vi "SimpleRobot_Dynamics_RevA.vi"(0 "x0":dbl, 1 "Wind Speed":dbl, 2 "Wind Direction":dbl, 5 "x1":dbl, 7 "y0":dbl, 9 "y1":dbl, 11 "Velocity":dbl, 12 "Direction":dbl, 13 "DeltaT (timestep)":dbl) -> (4 "x 2":dbl, 6 "y 2":dbl, 10 "Direction 2":dbl, 15 "Boat Velocity Out":dbl)   [LabVIEW 2012]
doc: "This subVI produces simple simulated robot dynamics.\nYou will need to replace it with a better simulation of your robot's dynamics"
panel:
  out "atan2(y,x)":dbl
  # "This VI calculates the Robot dynamics from frame to frame (one frame equals one time step)"
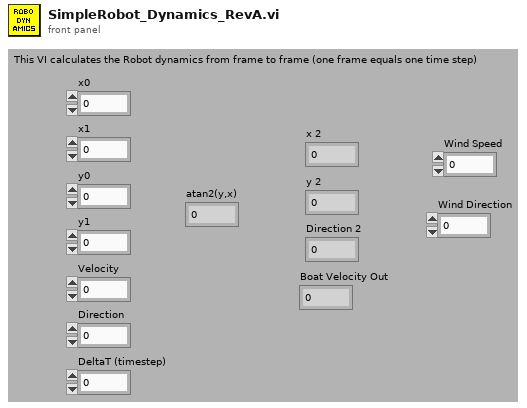
[diagram p1: front panel]
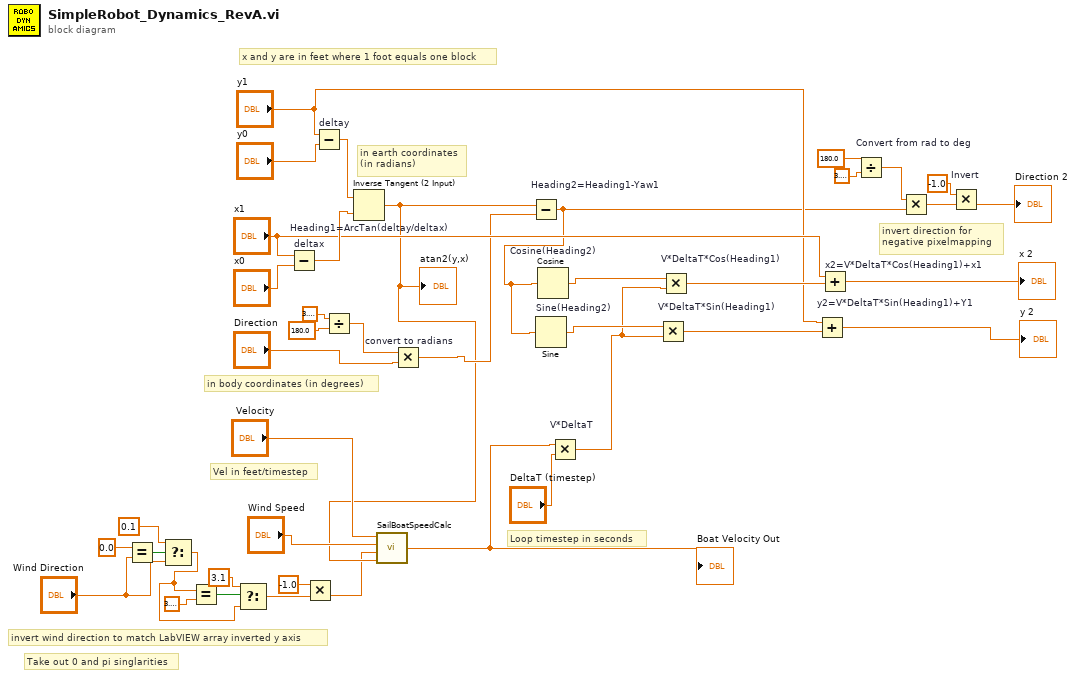
[diagram p0: block diagram]
diagram:
  # "Take out 0 and pi singlarities"
  # "invert wind direction to match LabVIEW array inverted y axis"
  # "invert direction for \nnegative pixelmapping"
  # "Loop timestep in seconds"
  # "x and y are in feet where 1 foot equals one block"
  # "Vel in feet/timestep"
  # "in earth coordinates\n(in radians)"
  # "in body coordinates (in degrees)"
  n1 = Equal?(x=0.0, y="Wind Direction") -> (x = y?=w9:bool)
  n2 = Select(t=0.1, s=w9, f="Wind Direction") -> (s? t:f=w1:dbl)
  n3 = Equal?(x=w1, y=3.141592653589793) -> (x = y?=w3:bool)
  n4 = Select(t=3.1, s=w3, f=w1) -> (s? t:f=w5:dbl)
  n5 = Subtract "deltax"(x="x1", y="x0") -> (x-y=w38:dbl)
  n6 = Multiply(x=-1.0, y=w5) -> (x*y=w11:dbl)
  n7 = Subtract "deltay"(x="y1", y="y0") -> (x-y=w39:dbl)
  n8 = Divide(x=3.141592653589793, y=180.0) -> (x/y=w27:dbl)
  n9 = Inverse Tangent (2 Input) "Heading1=ArcTan(deltay/deltax)"(1:w38, 2:w39) -> (0:w13:dbl)
  "atan2(y,x)" <- w13
  n10 = call "SailBoatSpeedCalc.vi"("Boat Direction"=w13, "Wind Direction (Rad global coordinates)"=w11, "Wind Speed"="Wind Speed", "Velocity Desired In"="Velocity") -> ("Boat Velocity Out"=w18:dbl)
  "Boat Velocity Out" <- w18
  n11 = Multiply "convert to radians"(x=w27, y="Direction") -> (x*y=w14:dbl)
  n12 = Subtract "Heading2=Heading1-Yaw1"(x=w13, y=w14) -> (x-y=w15:dbl)
  n13 = Sine "Sine(Heading2)"(x=w15) -> (sin(x)=w36:dbl)
  n14 = Cosine "Cosine(Heading2)"(x=w15) -> (cos(x)=w37:dbl)
  n15 = Multiply "V*DeltaT"(x=w18, y="DeltaT (timestep)") -> (x*y=w35:dbl)
  n16 = Multiply "V*DeltaT*Sin(Heading1)"(x=w36, y=w35) -> (x*y=w12:dbl)
  n17 = Multiply "V*DeltaT*Cos(Heading1)"(x=w37, y=w35) -> (x*y=w34:dbl)
  n18 = Add "y2=V*DeltaT*Sin(Heading1)+Y1"(x="y1", y=w12) -> (x+y=→"y 2":dbl)
  n19 = Add "x2=V*DeltaT*Cos(Heading1)+x1"(x="x1", y=w34) -> (x+y=→"x 2":dbl)
  n20 = Divide "Convert from rad to deg"(x=180.0, y=3.141592653589793) -> (x/y=w23:dbl)
  n21 = Multiply(x=w23, y=w15) -> (x*y=w20:dbl)
  n22 = Multiply "Invert"(x=-1.0, y=w20) -> (x*y=→"Direction 2":dbl)
